vi "Tank.vi"() -> ()   [LabVIEW 2016]
uses:
  Pathfinder-Lib/VIs/Waypoint.ctl
  Pathfinder-Lib/Pathfinder.lvlib
panel:
  in  "Tab Control":enum32{"Primary Path", "Tank Position"}(tab)=enum."Tank Position"
  out "Path":T1(graph)
  out "Position":cluster{dbl[], dbl[]}[](graph)
  out "error out":errorcluster
  in  "wheelbase_width":dbl=24.0
  in  "sample_count":i32=1000
  in  "dt":dbl=0.001
  in  "max_jerk":dbl=60.0
  in  "max_acceleration":dbl=10.0
  in  "max_velocity":dbl=15.0
  in  "path":T2[](array[typedef])=[{"x"=12.0, "y"=60.0, "angle"=0.0}, {"x"=132.0, "y"=125.0, "angle"=60.0}]
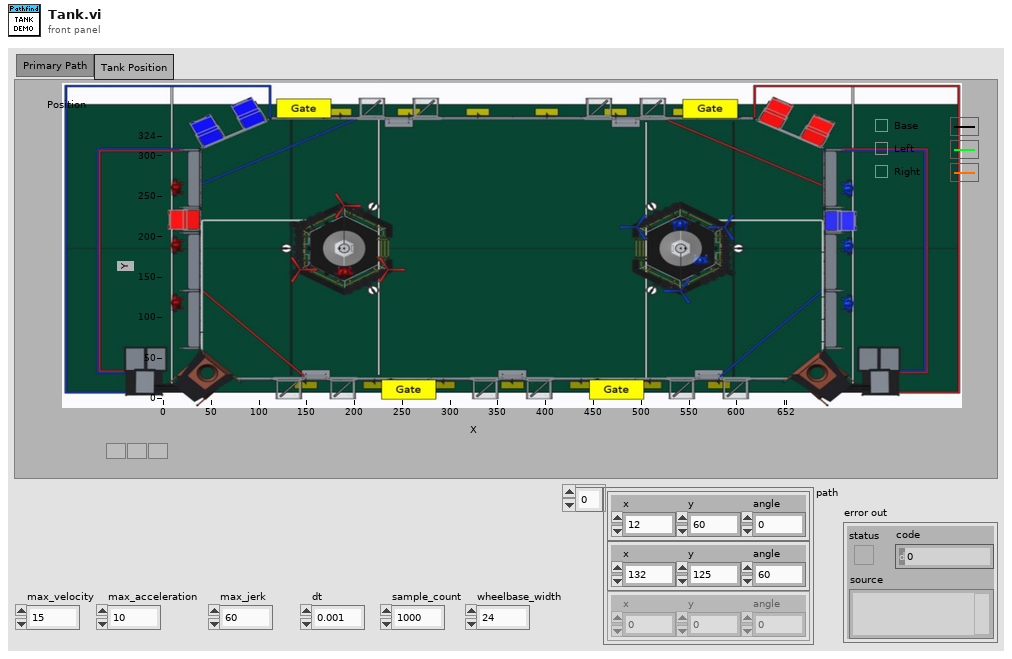
[diagram p1: front panel]
types:
  T1 = cluster{"position":dbl, "velocity":dbl, "acceleration":dbl, "jerk":dbl, "heading":dbl}[]
  T2 = typedef "Pathfinder.lvlib/Waypoint.ctl" = cluster{"x":dbl, "y":dbl, "angle":dbl}
  T3 = typedef "Pathfinder.lvlib/Segment.ctl" = cluster{"dt":dbl, "x":dbl, "y":dbl, "position":dbl, "velocity":dbl, "acceleration":dbl, "jerk":dbl, "heading":dbl}
  T4 = cluster{"position":dbl, "velocity":dbl, "acceleration":dbl, "jerk":dbl, "heading":dbl}
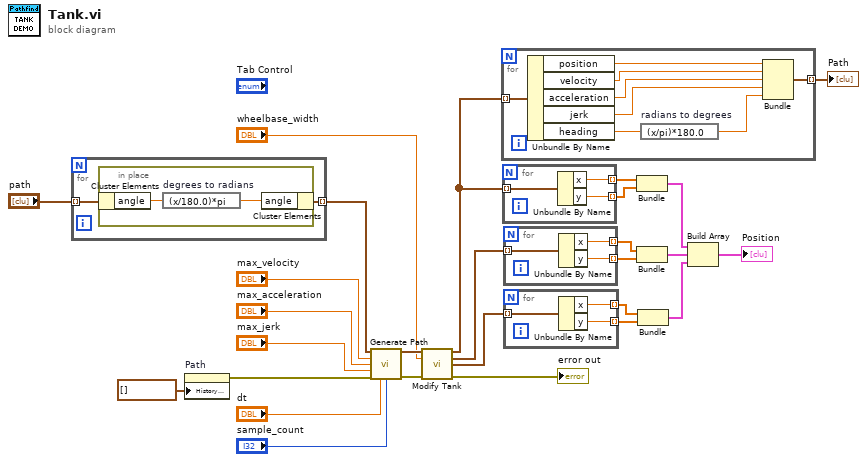
[diagram p0: block diagram]
diagram:
  n1 = for {
    tunnel: "path" -> [w29] mode=indexing
    tunnel: [w28] -> w2 mode=indexing
    n2 = in-place {
      n3 = in-place-cluster #1(w29) -> ("angle"=w31:dbl)
      n4 = expression code="(x/180.0)*pi" "degrees to radians"(w31) -> (w30:dbl)
      n5 = in-place-cluster #1("angle"=w30) -> (w28:T2)
    }
  }
  n6 = property on="Path" class="WFChart (strict)"("History Data"=T1 []) -> (error out=w4:errorcluster)  [unwired: 2 in, 1 out]
  n7 = call "Generate Path.vi"("path"=w2, "max_velocity"="max_velocity", "max_acceleration"="max_acceleration", "max_jerk"="max_jerk", "error in"=w4, "dt (.001)"="dt", "sample_count (100000)"="sample_count") -> ("Segments"=w27:T3[], "error out"=w23:errorcluster)  [unwired: 7 in]
  n8 = call "Modify Tank.vi"("Original"=w27, "wheelbase_width"="wheelbase_width", "error in"=w23) -> ("original"=w9:T3[], "left"=w18:T3[], "right"=w17:T3[], "error out"=→"error out":errorcluster)  [unwired: 9 in]
  n9 = for {
    tunnel: w9 -> [w39] mode=indexing
    tunnel: [w33] -> w19 mode=indexing
    n10 = Unbundle By Name(w39) -> ("position"=w38:dbl, "velocity"=w37:dbl, "acceleration"=w36:dbl, "jerk"=w35:dbl, "heading"=w34:dbl)
    n11 = expression code="(x/pi)*180.0" "radians to degrees"(w34) -> (w32:dbl)
    n12 = Bundle("position"=w38, "velocity"=w37, "acceleration"=w36, "jerk"=w35, "heading"=w32) -> (w33:T4)  [unwired: 1 in]
  }
  "Path" <- w19
  n13 = for {
    tunnel: w9 -> [w42] mode=indexing
    tunnel: [w41] -> w8 mode=indexing
    tunnel: [w40] -> w7 mode=indexing
    n14 = Unbundle By Name(w42) -> ("x"=w41:dbl, "y"=w40:dbl)
  }
  n15 = for {
    tunnel: w18 -> [w45] mode=indexing
    tunnel: [w44] -> w16 mode=indexing
    tunnel: [w43] -> w15 mode=indexing
    n16 = Unbundle By Name(w45) -> ("x"=w44:dbl, "y"=w43:dbl)
  }
  n17 = for {
    tunnel: w17 -> [w48] mode=indexing
    tunnel: [w47] -> w14 mode=indexing
    tunnel: [w46] -> w13 mode=indexing
    n18 = Unbundle By Name(w48) -> ("x"=w47:dbl, "y"=w46:dbl)
  }
  n19 = Bundle(w8, w7) -> (w6:cluster{dbl[], dbl[]})  [unwired: 1 in]
  n20 = Bundle(w16, w15) -> (w11:cluster{dbl[], dbl[]})  [unwired: 1 in]
  n21 = Bundle(w14, w13) -> (w12:cluster{dbl[], dbl[]})  [unwired: 1 in]
  n22 = Build Array(w6, w11, w12) -> (→"Position":cluster{dbl[], dbl[]}[])
